vi "GFITS_SelectArrData.vi"(10 "arr name":string) -> (0 "index":i32, 1 "subset?":bool, 2 "name out":string, 3 "comment":string)   [LabVIEW 2016]
uses:
  DBSHAND/private/vis/DatabaseHand_RefNum.ctl
panel:
  in  "Database RefNum in":T1
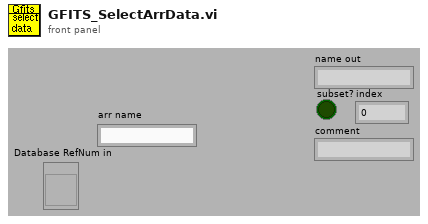
[diagram p1: front panel]
types:
  T1 = typedef "DatabaseHand_RefNum.ctl" = refnum<vi>
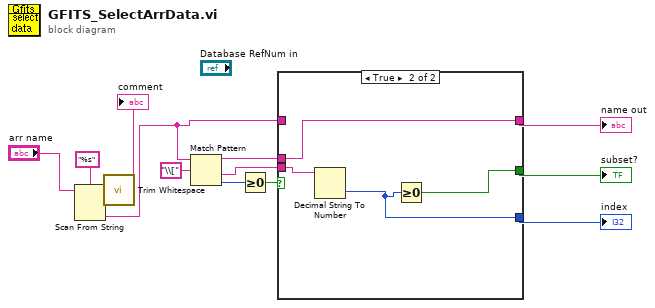
[diagram p0: block diagram]
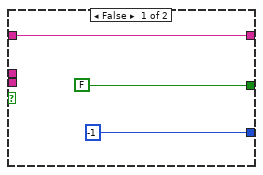
[diagram p2: hidden frame]
diagram:
  n1 = Scan From String(format string="%s", input string="arr name") -> (remaining string=w2:string, output 1=w3:string)  [unwired: 2 in, 3 out]
  n2 = call <vilib>:"Trim Whitespace.vi"("string"=w2) -> ("trimmed string"=→"comment":string)  [unwired: 1 in]
  n3 = Match Pattern(string=w3, regular expression="\\[") -> (before substring=w6:string, after substring=w7:string, offset past match=w12:i32)  [unwired: 2 out]
  n4 = Greater Or Equal To 0?(x=w12) -> (x >= 0?=w11:bool)
  n5 = case shown="True" w11 {
    tunnel: w3 -> [w16 _]
    tunnel: [w16 w19] -> w10
    tunnel: [FALSE w17] -> w9
    tunnel: [-1 w18] -> w8
    tunnel: w7 -> [_ w20]
    tunnel: w6 -> [_ w19]
    frame False {
    }
    frame True {
      n6 = Decimal String To Number(string=w20) -> (number=w18:i32)  [unwired: 3 out]
      n7 = Greater Or Equal To 0?(x=w18) -> (x >= 0?=w17:bool)
    }
  }
  "name out" <- w10
  "subset?" <- w9
  "index" <- w8
